vi "PFI-28000-Base_Read Response.vi"(0 "PFI-28000-Base in":refnum<class "PFI-28000-Base.lvclass">, 11 "error in (no error)":errorcluster) -> (4 "PFI-28000-Base out":refnum<class "PFI-28000-Base.lvclass">, 6 "Response":string, 8 "Timed Out":bool, 15 "error out":errorcluster)   [LabVIEW 2017, in "PFI-28000-Base.lvclass"]
uses:
  PFI-28000-Base.lvclass
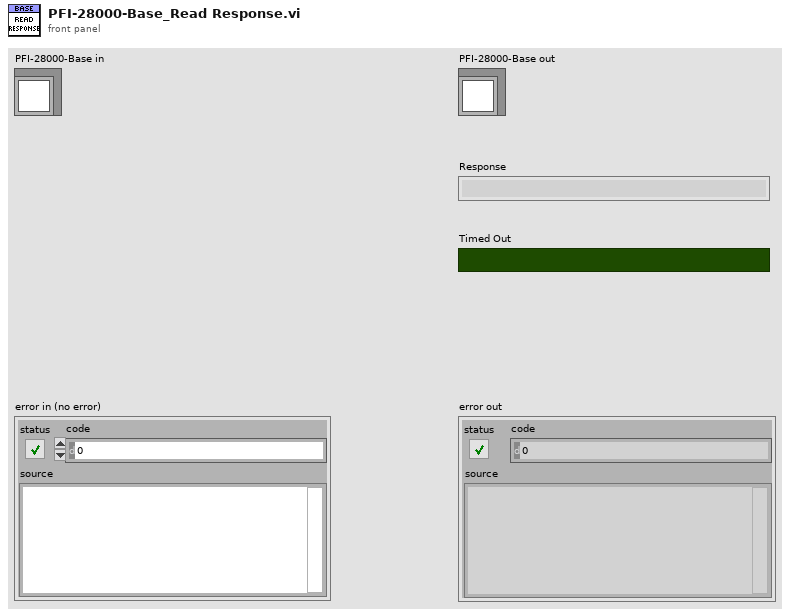
[diagram p1: front panel]
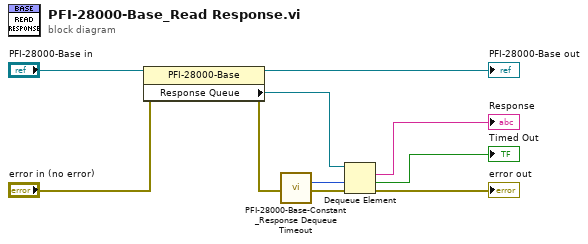
[diagram p0: block diagram]
diagram:
  n1 = property class="PFI-28000-Base"(reference="PFI-28000-Base in", error in="error in (no error)") -> (reference out=→"PFI-28000-Base out":refnum<class "PFI-28000-Base.lvclass">, error out=w3:errorcluster, "Response Queue"=w9:refnum<queue>)
  n2 = call "PFI-28000-Base-Constant_Response Dequeue Timeout.vi"() -> ("Timeout"=w8:i32)  [unwired: 15 in]
  n3 = Dequeue Element(queue=w9, timeout in ms (-1)=w8, error in (no error)=w3) -> (element=→"Response":string, timed out?=→"Timed Out":bool, error out=→"error out":errorcluster)  [unwired: 1 out]
